vi "call include vi script.vi"(8 "error in (no error)":errorcluster, 11 "state cluster":T1) -> (0 "error out":errorcluster)   [LabVIEW 2013, in "RT Temperature Controller.lvlib"]
uses:
  RT Temperature Controller.lvlib
  Controls/StateCluster.ctl
  <vilib>/NI/Tag Bus Data Framework/Configuration Editor/Classes/SystemConfigRepo/SystemConfigRepo.lvclass
  <vilib>/CEF_TreeControl/Node/NodeRef.ctl
  <vilib>/CEF_TreeControl/Node/NISE_CEF_Node.lvclass
  <vilib>/CEF_TreeControl/Node/UserEventRef.ctl
  <vilib>/CEF_TreeControl/Controls/EventCluster.ctl
  SplashScreen/splash screen.ctl
  SplashScreen/notifier data.ctl
  <vilib>/NI/Tag Bus Data Framework/Framework Configuration Classes/class cache/PL_class cache.lvlib
  <vilib>/CEF_TreeControl/NISE_CEF_TreeControl.lvlib
  SplashScreen/splash screen.lvlib
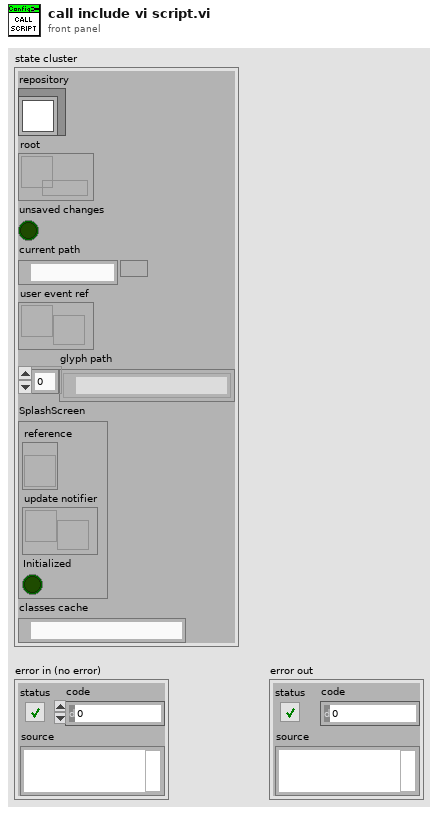
[diagram p1: front panel]
types:
  T1 = typedef "RT Temperature Controller.lvlib/StateCluster.ctl" = cluster{"repository":refnum<class "SystemConfigRepo.lvclass">, "root":T2, "unsaved changes":bool, "current path":path, "user event ref":T3, "glyph path":path[], "SplashScreen":T4, "classes cache":path}
  T2 = typedef "NISE_CEF_Node.lvclass/NodeRef.ctl" = refnum<data-value>
  T3 = typedef "NISE_CEF_Node.lvclass/UserEventRef.ctl" = refnum<user-event>
  T4 = typedef "RT Temperature Controller.lvlib/splash screen.lvlib/splash screen.ctl" = cluster{"reference":refnum<vi>, "update notifier":refnum<notifier>, "Initialized":bool}
  T5 = typedef "PL_class cache.lvlib/cache definition.ctl" = cluster{"configuration":T6, "class cache data":T7}
  T6 = typedef "PL_class cache.lvlib/cache search configuration.ctl" = cluster{"Search Paths":path[], "Folders to Exclude":string[], "full class list":path[]}
  T7 = typedef "PL_class cache.lvlib/cached class information.ctl" = cluster{"targets":T8[], "engines":T9[], "modules":T9[], "ignored class list":path[]}
  T8 = typedef "PL_class cache.lvlib/target class metadata.ctl" = cluster{"file name":string, "fully qualified name":string, "menu display name":string, "configuration class name":string}
  T9 = typedef "PL_class cache.lvlib/class metadata.ctl" = cluster{"file name":string, "fully qualified name":string, "menu display name":string, "configuration class":string, "instances allowed":i32, "supported targets":T10[]}
  T10 = typedef "TBM configuration.lvclass/Target Types.ctl" = enum16{"Windows", "Mac", "Linux", "Linux RT ARM", "VxWorks", "Pharlap", "Other", "Linux RT x64"}
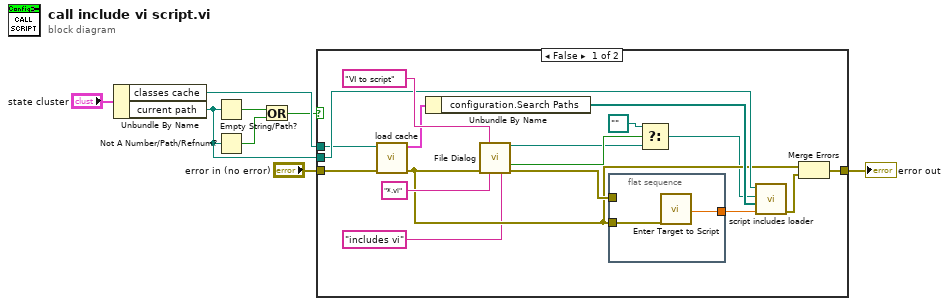
[diagram p0: block diagram]
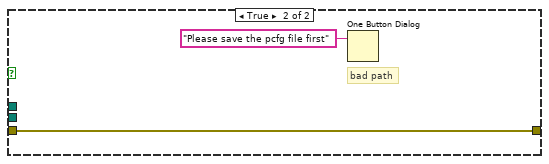
[diagram p2: hidden frame]
diagram:
  n1 = Unbundle By Name("state cluster") -> ("classes cache"=w6:path, "current path"=w5:path)
  n2 = Empty String/Path?(string/path=w5) -> (empty?=w3:bool)
  n3 = Not A Number/Path/Refnum?(number/path/refnum=w5) -> (NaN/Path/Refnum?=w2:bool)
  n4 = Or(x=w3, y=w2) -> (x .or. y?=w4:bool)
  n5 = case shown="False" w4 {
    tunnel: w5 -> [w22 _]
    tunnel: w6 -> [w19 _]
    tunnel: "error in (no error)" -> [w18 w28]
    tunnel: [w16 w28] -> w8
    frame False {
      n6 = call <vilib>:"load cache.vi"("error in"=w18, "cache path"=w19) -> ("error out"=w14:errorcluster, "cache"=w23:T5)  [unwired: 8 in]
      n7 = Unbundle By Name(w23) -> ("configuration.Search Paths"=w21:path[])
      n8 = call "File Dialog"("prompt"="VI to script", "error in"=w14, "pattern (all files)"="*.vi", "pattern label"="includes vi") -> ("selected path"=w11:path, "cancelled"=w12:bool, "error out"=w15:errorcluster)  [unwired: 8 in, 1 out]
      n9 = flat-sequence {
        tunnel: [w27] -> w20
        tunnel: w15 -> [_]
        tunnel: w14 -> [w26]
        frame #0 {
          n10 = call "Enter Target to Script"("error in (no error)"=w26) -> ("Target Number (0)"=w27:dbl)  [unwired: 16 in, 2 out]
        }
      }
      n11 = Select(t=path "", s=w12, f=w11) -> (s? t:f=w13:path)
      n12 = call <vilib>:"script includes loader.vi"("target"=w20, "Plugin Search Paths"=w21, "vi path (blank=new)"=w13, "cfg file path"=w22) -> ("error out"=w17:errorcluster)  [unwired: 7 in]
      n13 = Merge Errors(w14, w17) -> (w16:errorcluster)
    }
    frame True {
      # "bad path"
      n14 = One Button Dialog(message="Please save the pcfg file first") -> ()  [unwired: 1 in, 1 out]
    }
  }
  "error out" <- w8
